vi "CB Feed Forward.vi"(9 "R":T1, 10 "Q":T1, 11 "State Space Model":T2) -> (3 "Feed Forward":T1)   [LabVIEW 2020]
uses:
  <vilib>/Analysis/Matrix/Datatypes/RealMatrix.ctl
  CB State Space.ctl
  <vilib>/Analysis/7linalg.llb/Real Transpose Matrix.vi
  <vilib>/Analysis/baseanly.llb/Real A x B.vi
  <vilib>/Analysis/_algsub.llb/Real PseudoInverse Matrix.vi
  <vilib>/Analysis/Matrix/Numeric/Add/Add - RM,RM.vi
  <vilib>/Analysis/NI_AALPro.lvlib
  <vilib>/Analysis/NI_AALBase.lvlib
  <vilib>/Analysis/Matrix/NI_Matrix.lvlib
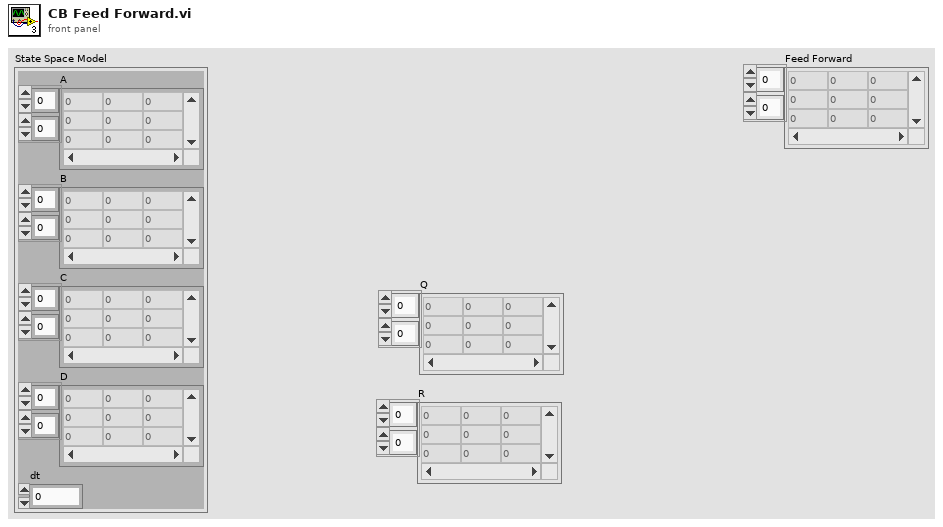
[diagram p1: front panel]
types:
  T1 = typedef "NI_Matrix.lvlib/RealMatrix.ctl" = dbl[][]
  T2 = typedef "CB State Space.ctl" = cluster{"A":T1, "B":T1, "C":T1, "D":T1, "dt":dbl}
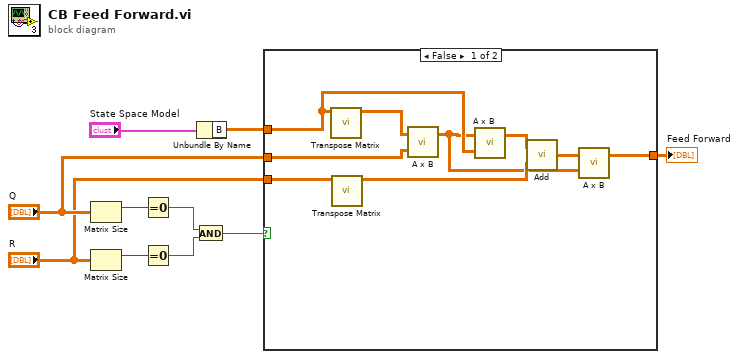
[diagram p0: block diagram]
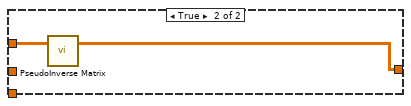
[diagram p2: hidden frame]
diagram:
  n1 = Matrix Size(0:"Q") -> (1:w10:i32)  [unwired: 1 out]
  n2 = Matrix Size(0:"R") -> (1:w9:i32)  [unwired: 1 out]
  n3 = Equal To 0?(x=w10) -> (x = 0?=w8:bool)
  n4 = Equal To 0?(x=w9) -> (x = 0?=w7:bool)
  n5 = And(x=w8, y=w7) -> (x .and. y?=w6:bool)
  n6 = Unbundle By Name("State Space Model") -> ("B"=w4:T1)
  n7 = case shown="False" w6 {
    tunnel: w4 -> [w16 w21]
    tunnel: "Q" -> [w17 _]
    tunnel: "R" -> [w19 _]
    tunnel: [w11 w20] -> w1
    frame False {
      n8 = call-poly <vilib>:"Transpose Matrix.vi"("Input Matrix"=w16) -> ("Matrix Transpose"=w18:T1)  [unwired: 9 in, 1 out]
      n9 = call-poly <vilib>:"Transpose Matrix.vi"("Input Matrix"=w19) -> ("Matrix Transpose"=w14:T1)  [unwired: 9 in, 1 out]
      n10 = call-poly <vilib>:"A x B.vi"("B"=w17, "A"=w18) -> ("A x B"=w12:T1)  [unwired: 1 out]
      n11 = call-poly <vilib>:"A x B.vi"("B"=w16, "A"=w12) -> ("A x B"=w15:T1)  [unwired: 1 out]
      n12 = call-poly <vilib>:"Add.vi"("Real Matrix B"=w14, "Real Matrix A"=w15) -> ("A + B"=w13:T1)
      n13 = call-poly <vilib>:"A x B.vi"("B"=w12, "A"=w13) -> ("A x B"=w11:T1)  [unwired: 1 out]
    }
    frame True {
      n14 = call-poly <vilib>:"PseudoInverse Matrix.vi"("Input Matrix"=w21) -> ("PseudoInverse Matrix"=w20:T1)  [unwired: 1 in, 1 out]
    }
  }
  "Feed Forward" <- w1
